vi "Subvi for Tree.vi"(8 "lvl size":u32, 9 "dataptr":u32, 11 "refnum IN":refnum<file>) -> (0 "dataptr for next lv":u32, 1 "nchildren":u32, 3 "refnum OUT":refnum<file>)   [LabVIEW 2017, in "HEKAdat.lvclass"]
uses:
  HEKAdat.lvclass
panel:
  out "error out":errorcluster
  in  "error in":errorcluster
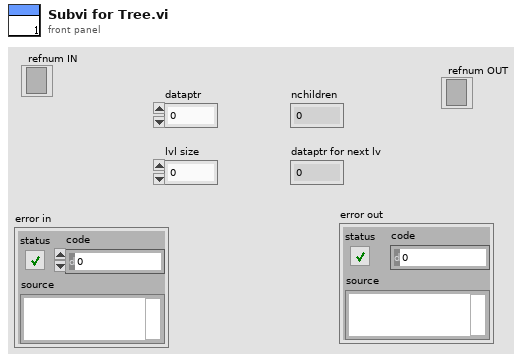
[diagram p1: front panel]
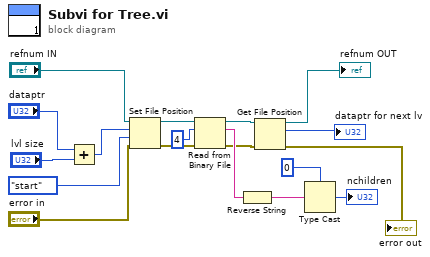
[diagram p0: block diagram]
diagram:
  n1 = Add(x="dataptr", y="lvl size") -> (x+y=w16:u32)
  n2 = Set File Position(offset (in bytes) (0)=w16, refnum="refnum IN", from (0:start)=enum16{"start", "end", "current"}."start", error in="error in") -> (refnum out=w15:refnum<file>, error out=w4:errorcluster)
  n3 = Read from Binary File(8:w4, 10:4 ("오프셋(0)"), 11:w15) -> (0:w9:errorcluster, 2:w13:string, 3:w8:refnum<file>)  [unwired: 3 in, 1 out]
  n4 = Reverse String(1:w13) -> (0:w12:string)
  n5 = Get File Position(4:w9, 7:w8) -> (0:→"error out":errorcluster, 2:→"dataptr for next lv":i64, 3:→"refnum OUT":refnum<file>)
  n6 = Type Cast(type=u32 0, x=w12) -> (*(type *) &x=→"nchildren":u32)
